vi "Set Item Resource String.vi"(7 "ItemName (ASCII)":string, 8 "error in (no error)":errorcluster, 9 "Text (UTF-16)":string, 10 "Language":i32, 11 "Menu Data in":refnum<class "Menu Data.lvclass">) -> (0 "error out":errorcluster, 3 "Menu Data out":refnum<class "Menu Data.lvclass">)   [LabVIEW 2013, in "SET Project Data.lvlib" / "Menu Data.lvclass"]
uses:
  Menu Data.lvclass
  Menu Data.lvclass/Menu Data.ctl
  Resource Data Class/Resource Data.lvclass
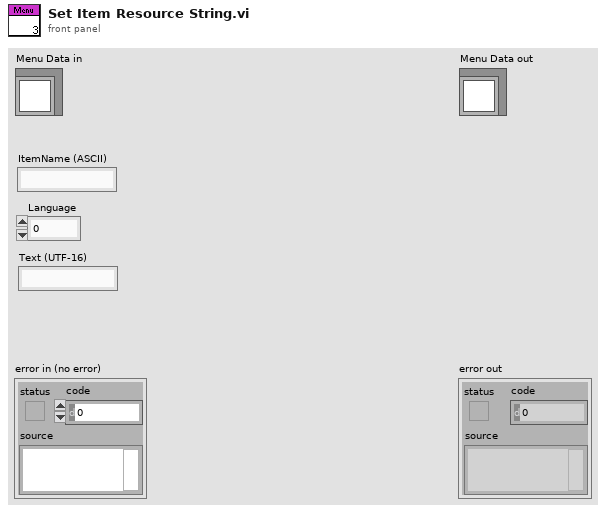
[diagram p1: front panel]
types:
  T1 = typedef "SET Project Data.lvlib/ProjFile_Resource Entry.ctl" = cluster{"RID":string, "Tag":string, "Strings [] (UTF-16)":string[], "Shared?":bool}
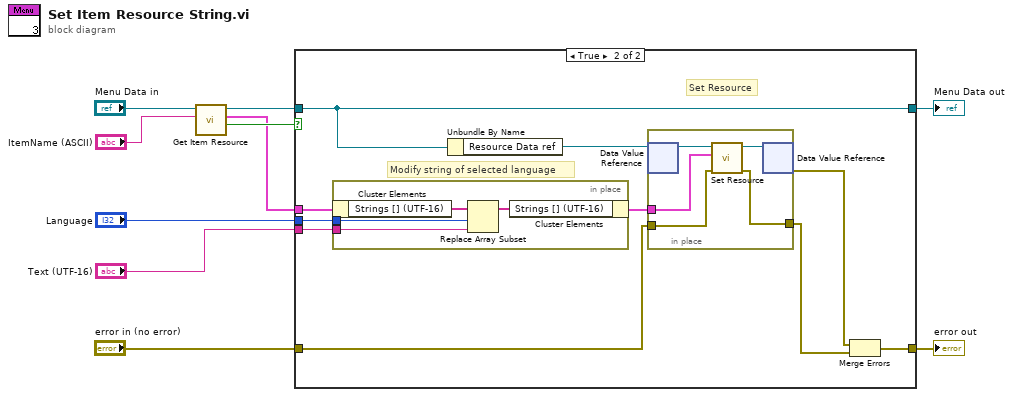
[diagram p0: block diagram]
diagram:
  n1 = call "Get Item Resource.vi"("ItemName"="ItemName (ASCII)", "Menu Data in"="Menu Data in") -> ("Found?"=w5:bool, "Resource"=w4:T1, "Menu Data out"=w7:refnum<class "Menu Data.lvclass">)  [unwired: 5 in, 2 out]
  n2 = case shown="True" w5 {
    tunnel: [w11 w14] -> w10
    tunnel: [w12 w18] -> w9
    tunnel: w7 -> [w12 w18]
    tunnel: w4 -> [_ w22]
    tunnel: "Language" -> [_ w21]
    tunnel: "Text (UTF-16)" -> [_ w20]
    tunnel: "error in (no error)" -> [w11 w16]
    frame False {
    }
    frame True {
      # "Set Resource"
      # "Modify string of selected language"
      n3 = in-place {
        in-place-border: w21 -> [w29]
        in-place-border: w20 -> [w28]
        n4 = in-place-cluster #1(w22) -> ("Strings [] (UTF-16)"=w31:string[])
        n5 = Replace Array Subset(array=w31, new element=w28, index=w29) -> (w30:string[])
        n6 = in-place-cluster #1("Strings [] (UTF-16)"=w30) -> (w19:T1)
      }
      n7 = Unbundle By Name(w18) -> ("Resource Data ref"=w17:refnum<data-value>)
      n8 = in-place {
        in-place-border: w19 -> [w26]
        in-place-border: w16 -> [w24]
        in-place-border: [w23] -> w15
        n9 = in-place-dvr #2(w17) -> (w27:refnum<class "Resource Data.lvclass">)  [unwired: 1 out]
        n10 = call "Set Resource.vi"("error in (no error)"=w24, "Resource"=w26, "LangFile in"=w27) -> ("error out"=w23:errorcluster, "LangFile out"=w25:refnum<class "Resource Data.lvclass">)  [unwired: 7 in]
        n11 = in-place-dvr #2(w25) -> (w13:errorcluster)  [unwired: 1 out]
      }
      n12 = Merge Errors(w13, w15) -> (w14:errorcluster)
    }
  }
  "error out" <- w10
  "Menu Data out" <- w9
